vi "FTW-Endpoint-Bind.vi"(0 "FTW Endpoint":refnum<class "FTW-Endpoint-TCP.lvclass">, 5 "Endpoint Address":string, 7 "Requested Identity":string, 11 "error in":errorcluster) -> (4 "FTW Endpoint out":refnum<class "FTW-Endpoint-TCP.lvclass">, 6 "Actual Endpoint Address":string, 8 "Actual Identity":string, 15 "error out":errorcluster)   [LabVIEW 2015, in "FTW-Endpoint-TCP.lvclass"]
uses:
  FTW-Endpoint-TCP.lvclass
  FTW-Endpoint-TCP.lvclass/FTW-Endpoint-TCP.ctl
panel:
  # "Inputs"
  # "Outputs"
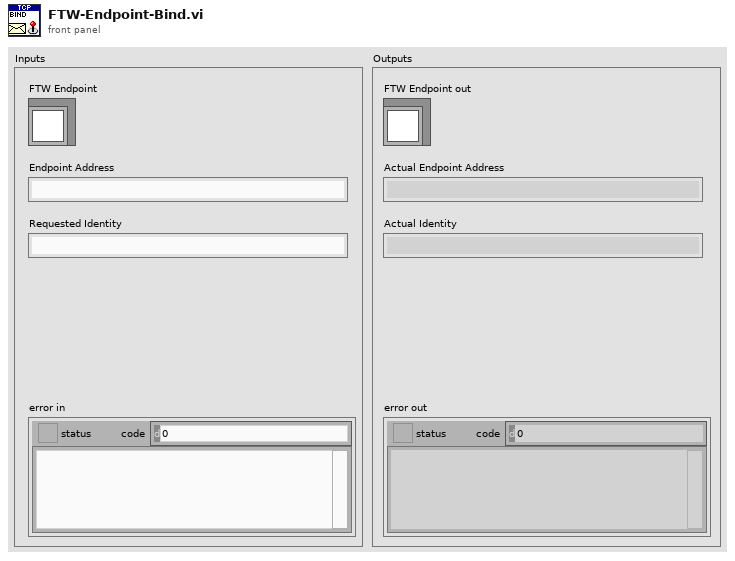
[diagram p1: front panel]
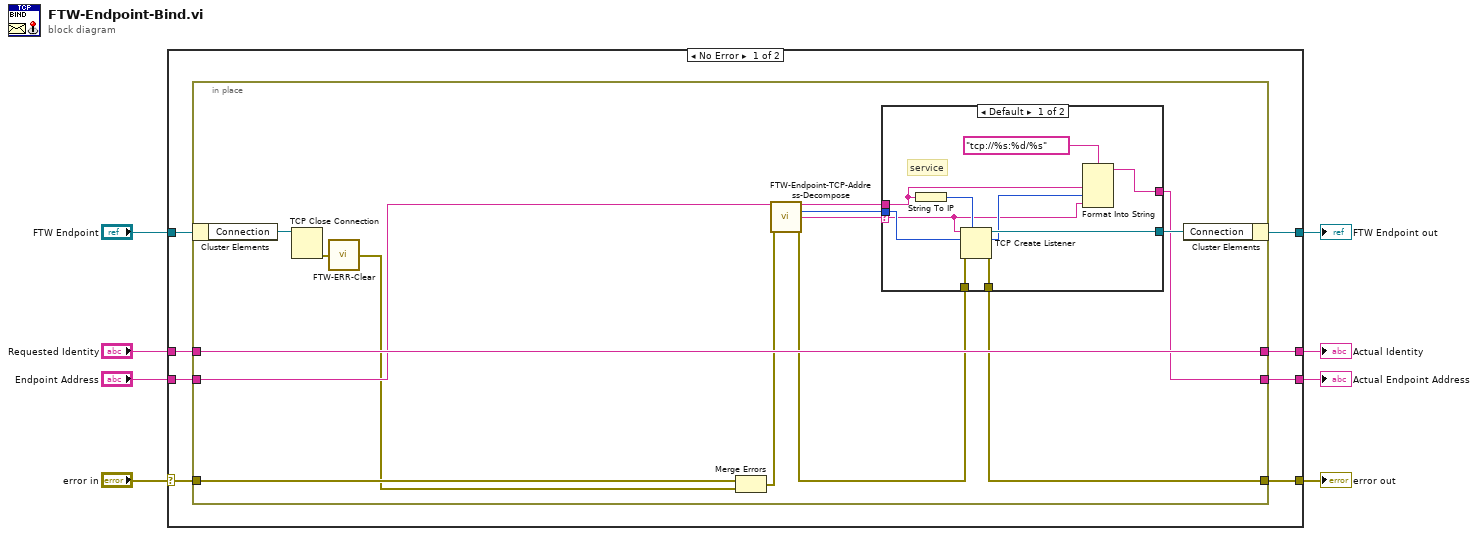
[diagram p0: block diagram]
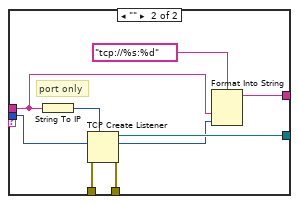
[diagram p2: hidden frame]
diagram:
  n1 = case shown="No Error" "error in" {
    selector: "error in" -> [w14 w51]
    tunnel: [w10 w51] -> w8
    tunnel: [w11 w50] -> w6
    tunnel: "FTW Endpoint" -> [w16 w50]
    tunnel: "Requested Identity" -> [w15 _]
    tunnel: "Endpoint Address" -> [w13 _]
    tunnel: [w12 _] -> w2
    tunnel: [w9 _] -> w1
    frame No Error {
      n2 = in-place {
        in-place-border: w15 -> [w29]
        in-place-border: w14 -> [w25]
        in-place-border: [w26] -> w10
        in-place-border: w13 -> [w23]
        in-place-border: [w18] -> w12
        in-place-border: [w29] -> w9
        n3 = in-place-cluster #1(w16) -> ("Connection"=w30:refnum<k5>)
        n4 = TCP Close Connection(connection ID=w30) -> (error out=w28:errorcluster)  [unwired: 2 in, 1 out]
        n5 = call "FTW-ERR-Clear.vi"("error to snuff"=w28) -> ("no error"=w21:errorcluster)
        n6 = Merge Errors(w25, w21) -> (w22:errorcluster)
        n7 = call "FTW-Endpoint-TCP-Address-Decompose.vi"("Endpoint Address"=w23, "error in"=w22) -> ("Domain"=w19:string, "Port"=w20:u16, "Service Name"=w17:string, "error out"=w24:errorcluster)  [unwired: 10 in]
        n8 = case shown="Default" w17 {
          selector: w17 -> [w31 _]
          tunnel: [w40 w49] -> w27
          tunnel: [w39 w48] -> w26
          tunnel: w24 -> [w38 w47]
          tunnel: w20 -> [w33 w41]
          tunnel: w19 -> [w34 w42]
          tunnel: [w36 w43] -> w18
          frame Default {
            # "service"
            n9 = String To IP(1:w34) -> (0:w35:u32)
            n10 = TCP Create Listener(7:w35, 8:w38, 10:w33, 11:w31) -> (0:w39:errorcluster, 2:w32:u16, 3:w40:refnum<k5>)  [unwired: 1 in]
            n11 = Format Into String(format string="tcp://%s:%d/%s" ("input string"), w34, w32, w31) -> (resulting string=w36:string)  [unwired: 2 in, 1 out]
          }
          frame "" {
            # "port only"
            n12 = String To IP(1:w42) -> (0:w46:u32)
            n13 = TCP Create Listener(7:w46, 8:w47, 10:w41) -> (0:w48:errorcluster, 2:w44:u16, 3:w49:refnum<k5>)  [unwired: 2 in]
            n14 = Format Into String(format string="tcp://%s:%d" ("input string"), w42, w44) -> (resulting string=w43:string)  [unwired: 2 in, 1 out]
          }
        }
        n15 = in-place-cluster #1("Connection"=w27) -> (w11:refnum<class "FTW-Endpoint-TCP.lvclass">)
      }
    }
    frame Error {
    }
  }
  "error out" <- w8
  "FTW Endpoint out" <- w6
  "Actual Endpoint Address" <- w2
  "Actual Identity" <- w1
